vi "Get String Control Terminal.vi"(8 "error in (no error)":errorcluster, 11 "String Control in":refnum<vi>) -> (0 "error out":errorcluster, 2 "Terminal":refnum<vi>, 3 "String Control out":refnum<vi>)   [LabVIEW 2019, in "VI Scripting Utilities.lvlib"]
uses:
  VI Scripting Utilities.lvlib
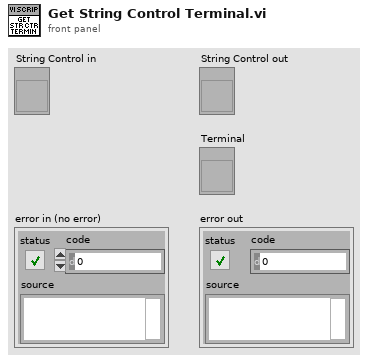
[diagram p1: front panel]
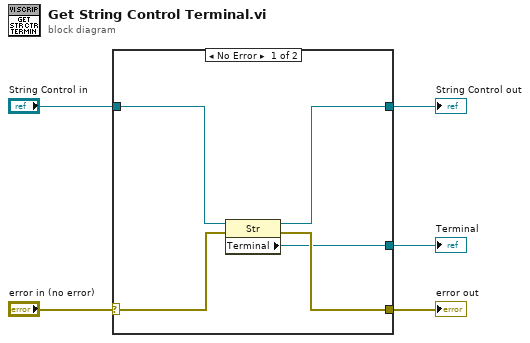
[diagram p0: block diagram]
diagram:
  n1 = case shown="No Error" "error in (no error)" {
    selector: "error in (no error)" -> [w6 w11]
    tunnel: [w10 w11] -> w5
    tunnel: [w9 w12] -> w4
    tunnel: [w8 _] -> w3
    tunnel: "String Control in" -> [w7 w12]
    frame No Error {
      n2 = property class="Str"(reference=w7, error in=w6) -> (reference out=w9:refnum<vi>, error out=w10:errorcluster, "Terminal"=w8:refnum<vi>)
    }
    frame Error {
    }
  }
  "error out" <- w5
  "String Control out" <- w4
  "Terminal" <- w3
